vi "Match Messages.vi"(8 "error in (no error)":errorcluster, 11 "RemoteControl in":refnum<class "RemoteControl.lvclass">) -> (0 "error out":errorcluster, 2 "Match":bool, 3 "RemoteControl out":refnum<class "RemoteControl.lvclass">)   [LabVIEW 2019, in "RemoteControl.lvclass"]
uses:
  RemoteControl.lvclass
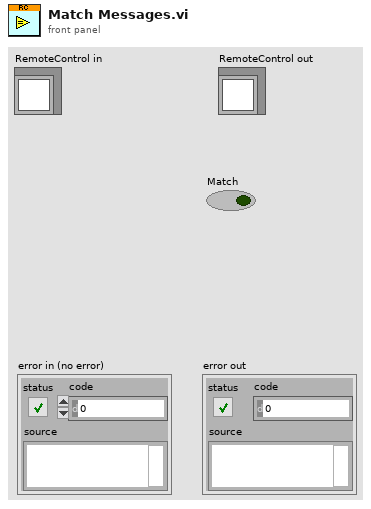
[diagram p1: front panel]
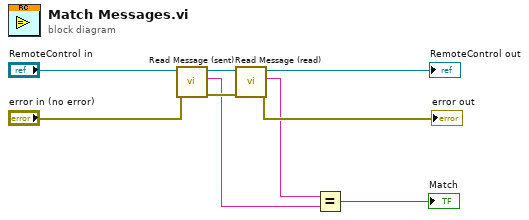
[diagram p0: block diagram]
diagram:
  n1 = call "Read Message (sent).vi"("error in (no error)"="error in (no error)", "RemoteControl in"="RemoteControl in") -> ("error out"=w6:errorcluster, "Command (Sent)"=w2:string, "RemoteControl out"=w9:refnum<class "RemoteControl.lvclass">)  [unwired: 5 in, 2 out]
  n2 = call "Read Message (read).vi"("error in (no error)"=w6, "RemoteControl in"=w9) -> ("error out"=→"error out":errorcluster, "Command (Read)"=w3:string, "RemoteControl out"=→"RemoteControl out":refnum<class "RemoteControl.lvclass">)  [unwired: 5 in, 2 out]
  n3 = Equal?(x=w3, y=w2) -> (x = y?=→"Match":bool)
